vi "Normalize Angle.vi"(10 "Input":dbl) -> (2 "Output":dbl)   [LabVIEW 2013, in "ProcessorHelperFunctions.lvlib"]
uses:
  ProcessorHelperFunctions.lvlib
panel:
  # "This VI takes an arbitrary angle and puts it between 0 and 360 degrees"
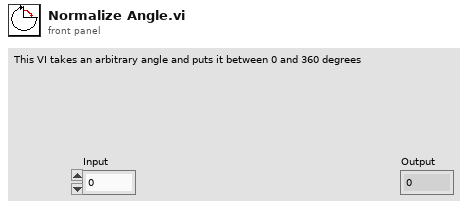
[diagram p1: front panel]
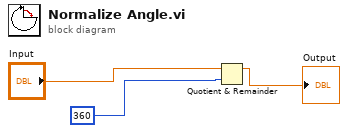
[diagram p0: block diagram]
diagram:
  n1 = Quotient & Remainder(x="Input", y=360) -> (x-y*floor(x/y)=→"Output":dbl)  [unwired: 1 out]
